vi "Enqueue if val.vi"(6 "read buffer":string, 8 "error in (no error)":errorcluster, 11 "Queue in":refnum<queue>) -> (0 "error out":errorcluster, 3 "Queue out":refnum<queue>)   [LabVIEW 2020]
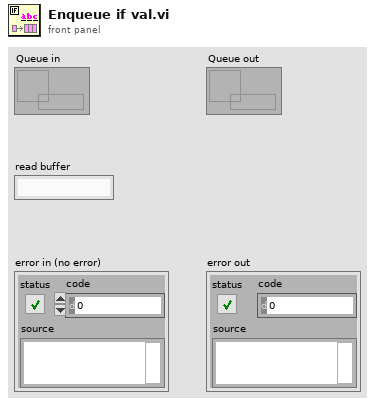
[diagram p1: front panel]
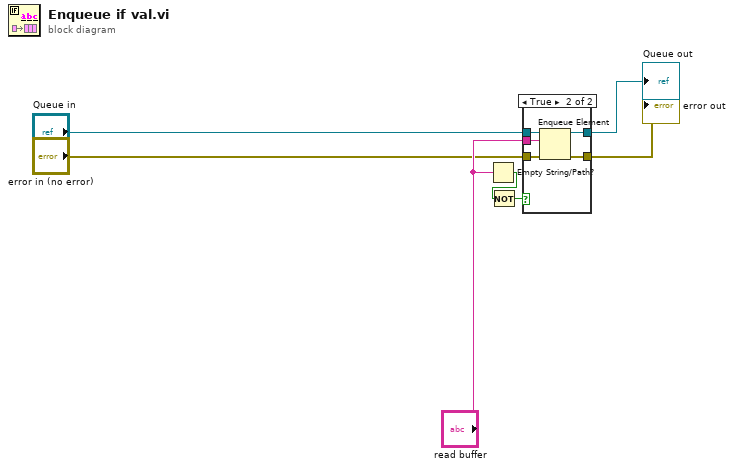
[diagram p0: block diagram]
diagram:
  n1 = Empty String/Path?(string/path="read buffer") -> (empty?=w5:bool)
  n2 = Not(x=w5) -> (.not. x?=w6:bool)
  n3 = case shown="True" w6 {
    tunnel: "read buffer" -> [_ w14]
    tunnel: "Queue in" -> [w9 w13]
    tunnel: "error in (no error)" -> [w8 w12]
    tunnel: [w8 w11] -> w3
    tunnel: [w9 w10] -> w4
    frame False {
    }
    frame True {
      n4 = Enqueue Element(queue=w13, element=w14, error in (no error)=w12) -> (queue out=w10:refnum<queue>, error out=w11:errorcluster)  [unwired: 1 in, 1 out]
    }
  }
  "Queue out" <- w4
  "error out" <- w3
